vi "Get_RegData_I32.vi"(8 "error in (no error)":errorcluster, 11 "Class in":refnum<class "IB_RegData_I32.lvclass">) -> (0 "error out":errorcluster, 2 "I32":i32, 3 "Class out":refnum<class "IB_RegData_I32.lvclass">)   [LabVIEW 2020, in "IB_RegData_I32.lvclass"]
uses:
  <vilib>/AppBuilder/IB_Classes/RegData/RegData_I32/IB_RegData_I32.lvclass
  <vilib>/AppBuilder/IB_Classes/RegData/RegData_I32/IB_RegData_I32.lvclass/IB_RegData_I32.ctl
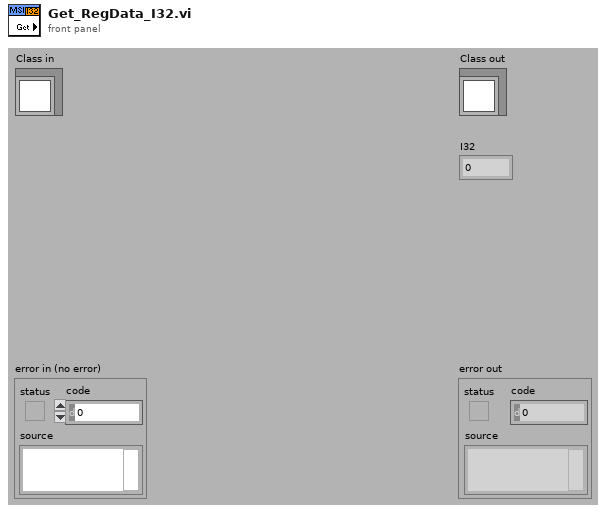
[diagram p1: front panel]
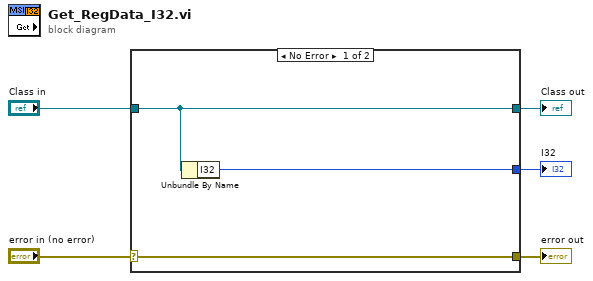
[diagram p0: block diagram]
diagram:
  n1 = case shown="No Error" "error in (no error)" {
    selector: "error in (no error)" -> [w8 w9]
    tunnel: [w8 w9] -> w4
    tunnel: [w7 w10] -> w2
    tunnel: "Class in" -> [w7 w10]
    tunnel: [w6 _] -> w1
    frame No Error {
      n2 = Unbundle By Name(w7) -> ("I32"=w6:i32)
    }
    frame Error {
    }
  }
  "error out" <- w4
  "Class out" <- w2
  "I32" <- w1
